vi "PMBus Read Word.vi"(4 "PEC":u8, 5 "pData":u16, 6 "CommandCode":u8, 7 "SlaveAddr":u8, 9 "PMBusIndex":i32, 10 "DevIndex":i32, 11 "DevType":i32) -> (2 "function return":i32, 3 "pData out":u16)   [LabVIEW 2010, in "ControlPMBus.lvlib"]
doc: "int WINAPI PMBus_ReadWord(int DevType,int DevIndex,int PMBusIndex,unsigned char SlaveAddr,unsigned char CommandCode, unsigned short *pData,unsigned char PEC);"
uses:
  ControlPMBus.lvlib
  ControlPMBus/Ginkgo_Driver.dll
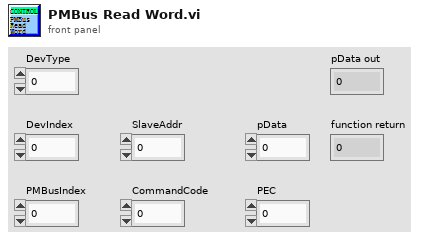
[diagram p1: front panel]
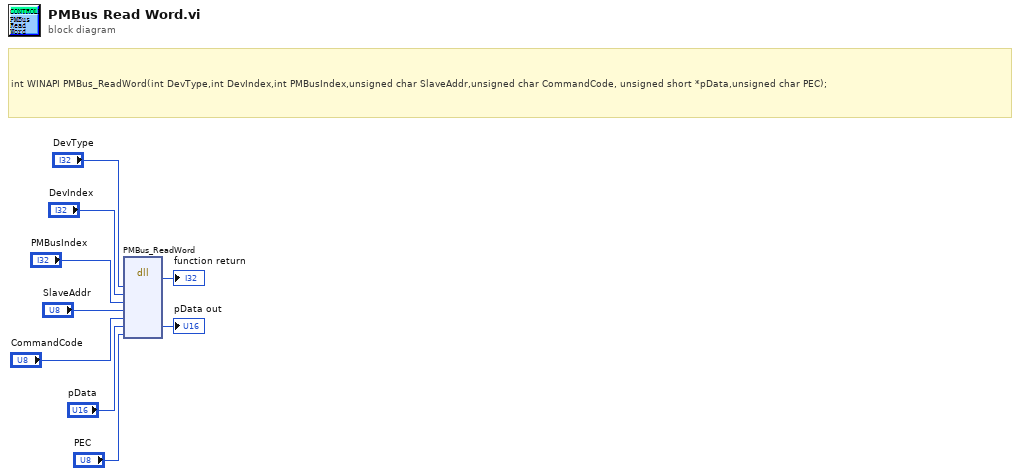
[diagram p0: block diagram]
diagram:
  # "int WINAPI PMBus_ReadWord(int DevType,int DevIndex,int PMBusIndex,unsigned char SlaveAddr,unsigned char CommandCode, unsigned short *pData,unsigned char PEC);"
  n1 = dll-call lib="E:/Project/vt_ginkgo/truck/Ginkgo Driver/vs2010/Ginkgo_USB-I2C&SPI&CAN_API_v2.0.3.3/lib/labview_32bit/ControlPMBus/Ginkgo_Driver.*" fn="PMBus_ReadWord"("DevType"="DevType", "DevIndex"="DevIndex", "PMBusIndex"="PMBusIndex", "SlaveAddr"="SlaveAddr", "CommandCode"="CommandCode", "pData"="pData", "PEC"="PEC") -> (→"function return":i32, "pData"=→"pData out":u16)  [unwired: 9 in, 2 out]
